vi "create test file.vi"() -> ()   [LabVIEW 2020]
panel:
  in  "file path":path
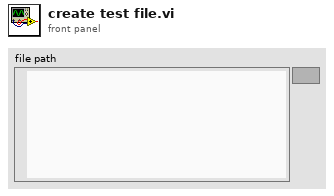
[diagram p1: front panel]
types:
  T1 = enum16{"open", "open or create", "create or replace", "create", "open (read-only)"}
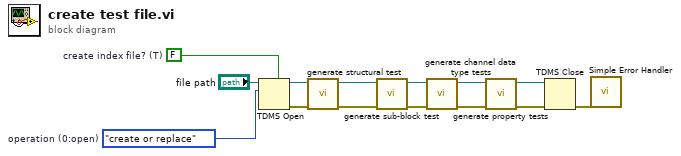
[diagram p0: block diagram]
diagram:
  w8 = T1."create or replace"  # operation (0:open)
  w10 = FALSE  # create index file? (T)
  n1 = TDMS Open(5:w10, 10:w8, 11:"file path") -> (0:w14:errorcluster, 3:w13:refnum<k34>)  [unwired: 4 in]
  n2 = call "generate structural test.vi"("error in (no error)"=w14, "Tdms File"=w13) -> ("error out"=w12:errorcluster, "Tdms File Out"=w6:refnum<k34>)  [unwired: 8 in]
  n3 = call "generate sub-block test.vi"("error in (no error)"=w12, "Tdms File"=w6) -> ("error out"=w7:errorcluster, "Tdms File Out"=w4:refnum<k34>)  [unwired: 8 in]
  n4 = call "generate channel data type tests.vi"("error in (no error)"=w7, "Tdms File"=w4) -> ("error out"=w5:errorcluster, "Tdms File Out"=w2:refnum<k34>)  [unwired: 8 in]
  n5 = call "generate property tests.vi"("error in (no error)"=w5, "Tdms File"=w2) -> ("error out"=w3:errorcluster, "Tdms File Out"=w1:refnum<k34>)  [unwired: 8 in]
  n6 = TDMS Close(8:w3, 11:w1) -> (0:w11:errorcluster)  [unwired: 1 out]
  n7 = call <vilib>:"Simple Error Handler.vi"("error in (no error)"=w11) -> ()  [unwired: 4 in, 5 out]
